vi "gloable.vi"() -> ()   [LabVIEW 2012]
panel:
  out "退出通知器":refnum<notifier>
  in  "事件注册引用句柄":refnum<event-registration>
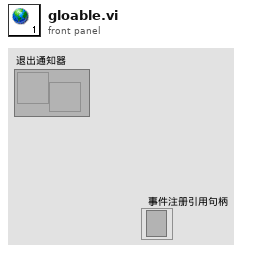
[diagram p1: front panel]
diagram:
